vi "Set homing parameters.vi"(11 "Acquisition data in":T1) -> (3 "Acquisition data out":T1)   [LabVIEW 2020, in "GUI.lvlib"]
uses:
  GUI.lvlib
  NI DAQ/Support/Continuous aquisition params.ctl
  NI DAQ/Support/Task list.ctl
  Support/Motor parameters.ctl
  NI DAQ/NI DAQ.lvlib
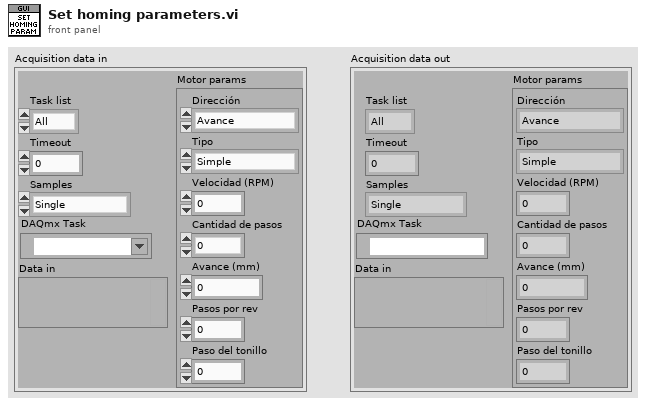
[diagram p1: front panel]
types:
  T1 = typedef "NI DAQ.lvlib/Continuous aquisition params.ctl" = cluster{"Task list":T2, "Timeout":i32, "Samples":enum16{"Single", "Multiple"}, "Data in":variant, "Motor params":T3, "DAQmx Task":refnum<k21>}
  T2 = typedef "NI DAQ.lvlib/Task list.ctl" = enum16{"All", "DO task", "DI task", "AO task", "AI task"}
  T3 = typedef "GUI.lvlib/Motor parameters.ctl" = cluster{"Dirección":enum16{"Avance", "Retroceso"}, "Tipo":enum16{"Simple", "Medio paso"}, "Velocidad (RPM)":dbl, "Cantidad de pasos":i32, "Avance (mm)":dbl, "Pasos por rev":dbl, "Paso del tonillo":dbl}
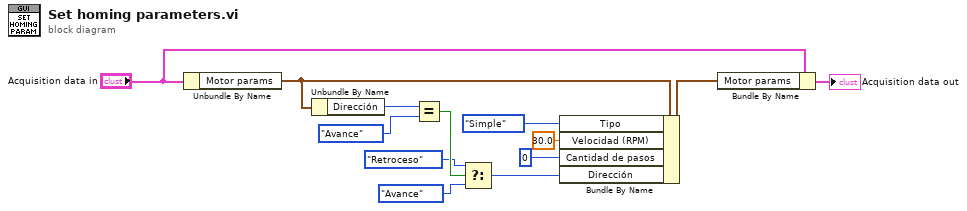
[diagram p0: block diagram]
diagram:
  n1 = Unbundle By Name("Acquisition data in") -> ("Motor params"=w11:T3)
  n2 = Unbundle By Name(w11) -> ("Dirección"=w6:enum16{"Avance", "Retroceso"})
  n3 = Equal?(x=w6, y=enum16{"Avance", "Retroceso"}."Avance" ("Dirección")) -> (x = y?=w4:bool)
  n4 = Select(t=enum16{"Avance", "Retroceso"}."Retroceso" ("Dirección"), s=w4, f=enum16{"Avance", "Retroceso"}."Avance" ("Dirección")) -> (s? t:f=w1:enum16{"Avance", "Retroceso"})
  n5 = Bundle By Name(cluster=w11, "Tipo"=enum16{"Simple", "Medio paso"}."Simple", "Velocidad (RPM)"=30.0, "Cantidad de pasos"=0, "Dirección"=w1) -> (w7:T3)
  n6 = Bundle By Name(cluster="Acquisition data in", "Motor params"=w7) -> (→"Acquisition data out":T1)
